vi "Linear Interpolation FtoD.vi"(5 "Interpolation Table(Xs,Ys)":dbl[][](array[numeric])=[[0.0, 0.0], [10.0, 65535.0]], 10 "Interp. X":dbl) -> (2 "Output Y":i32)   [LabVIEW 2009]
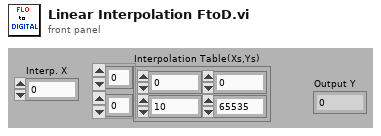
[diagram p1: front panel]
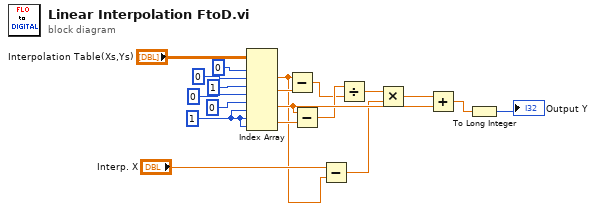
[diagram p0: block diagram]
diagram:
  w12 = 1 ("disabled index (col)")
  n1 = Index Array(array="Interpolation Table(Xs,Ys)", index (row) #1=0 ("index (row)"), index (col) #1=0 ("disabled index (col)"), index (row) #2=1 ("index (row)"), index (col) #2=0 ("disabled index (col)"), index (row) #3=0 ("index (row)"), index (col) #3=w12, index (row) #4=w12, index (col) #4=w12) -> (element #1=w5:dbl, element #2=w14:dbl, element #3=w8:dbl, element #4=w11:dbl)
  n2 = Subtract(x=w5, y=w14) -> (x-y=w3:dbl)
  n3 = Subtract(x=w8, y=w11) -> (x-y=w4:dbl)
  n4 = Subtract(x="Interp. X", y=w5) -> (x-y=w7:dbl)
  n5 = Divide(x=w4, y=w3) -> (x/y=w10:dbl)
  n6 = Multiply(x=w10, y=w7) -> (x*y=w9:dbl)
  n7 = Add(x=w9, y=w8) -> (x+y=w1:dbl)
  n8 = To Long Integer(number=w1) -> (32bit integer=→"Output Y":i32)
